vi "Close.vi"(8 "Error In":errorcluster, 11 "Sierra M100 In":refnum<visa-resource-name>) -> (0 "Error Out":errorcluster)   [LabVIEW 2012, in "Sierra-M100.lvlib"]
doc: "This VI safely closes communication with the mass flow controller (MFC) so other applications and VIs can communicate with the MFC as needed."
uses:
  Sierra-M100.lvlib
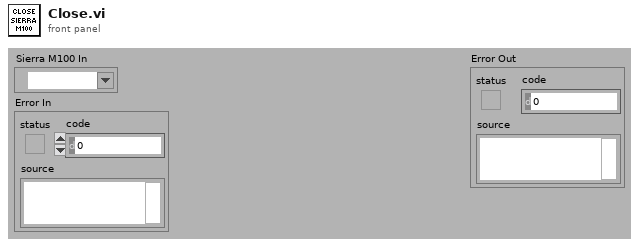
[diagram p1: front panel]
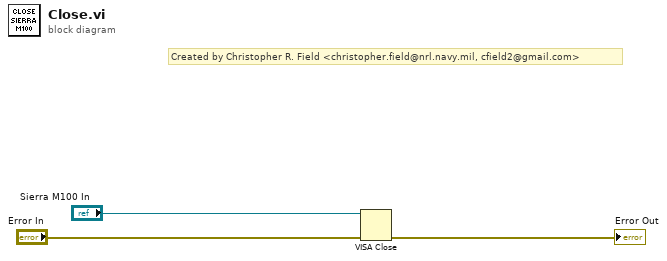
[diagram p0: block diagram]
diagram:
  # "Created by Christopher R. Field <christopher.field@nrl.navy.mil, cfield2@gmail.com>"
  n1 = VISA Close(VISA resource name="Sierra M100 In", error in (no error)="Error In") -> (error out=→"Error Out":errorcluster)
